vi "PhXP Settings Storage.vi"(6 "Set/Get(F)":bool, 8 "Error In":errorcluster, 10 "Variant Data in":variant, 11 "Settings List":T12) -> (0 "Error Out":errorcluster, 2 "Variant Data out":variant)   [LabVIEW 2019]
uses:
  Phasor Explorer Detector Parameters.ctl
  Phasor Explorer Gate Parameters.ctl
  Gate Type.ctl
  Phasor Explorer Decay Parameters.ctl
  IRF Model.ctl
  Phasor Explorer Phasor Parameters.ctl
  Phasor Calculation Type.ctl
  SEPL Type.ctl
  Phasor Explorer Display Parameters.ctl
  Type of Series.ctl
  Phasor Explorer Settings List.ctl
panel:
  in  "Parameter Tabs":T1(tab)=enum."Gates"
  in  "Phasor Explorer Display Parameters":T2={"# Points"=1000, "Ramp Type"=enum."Logarithmic", "Type of Series"=enum."1-Exp Decays", "Min tau"=1.0000000000000002e-12, "Max tau"=1.0000000000000001e-07, "Include 0"=FALSE, "Include Infinity"=FALSE} {"Min tau" min=0.0; "Max tau" min=0.0; "# Points" min=1 step=1}
  in  "f*":dbl[unit]=80000000.0 format="%#_5g"
  in  "tau*":dbl[unit]=1.9894367886486918e-09 format="%#_5g"
  in  "Phasor Explorer Phasor Parameters":T4={"Harmonic frequency"=80000000.0, "Use f* = 1/D Frequency"=FALSE, "Calibrated Phasor"=FALSE, "Calibration Lifetime"=1e-09, "Phasor Calculation"=enum."Direct Sum", "SEPL Type"=enum."UC", "# Gates"=1.0, "Square Gate Width"=1e-09, "Show Ticks"=FALSE} {"Square Gate Width" min=0.0; "# Gates" min=0.0; "Calibration Lifetime" min=0.0; "Harmonic frequency" min=0.0}
  in  "Phasor Explorer Decay Parameters":T7={"Lifetime"=3.0000000000000004e-09, "IRF Offset"=0.0, "IRF Period"=1.2500000000000001e-08, "Normalized Decays"=FALSE, "IRF Model"=enum."Dirac", "IRF Parameter 1"=0.0} {"Lifetime" min=0.0; "IRF Period" min=0.0}
  in  "Phasor Explorer Gate Parameters":T9={"First Gate Start"=0.0, "Use Gate Center"=FALSE, "Gate Width"=0.0, "Gate Step"=1.785714285714286e-09, "# Gates"=7.0, "Gate Type"=enum."Square", "Edge Width"=0.0, "Top Slope"=0.0, "Reversed Sawtooth?"=FALSE, "Analytical Computation"=FALSE, "Integration"=enum."Item 0", "Tolerance"=1.0, "# Steps"=1.0, "Type of User-defined Function"=enum."Gate", "Use Gate Step"=FALSE} {"# Steps" min=0.0; "Tolerance" min=0.0; "Top Slope" min=0.0; "Edge Width" min=0.0; "First Gate Start" format="%#_4g"; "Gate Step" min=0.0 format="%#_4g"; "# Gates" min=1.0 step=1.0; "Gate Width" min=0.0 format="%#_4g"}
  in  "Phasor Explorer Detector Parameters":T11={"Frames/Image"=0, "Gates/Frame"=1, "Bits/Frame"=1, "Multiplicity"=0, "Incident Signal"=0.0, "Poisson Signal"=FALSE} {"Frames/Image" min=1; "Multiplicity" min=0; "Bits/Frame" min=1; "Gates/Frame" min=1}
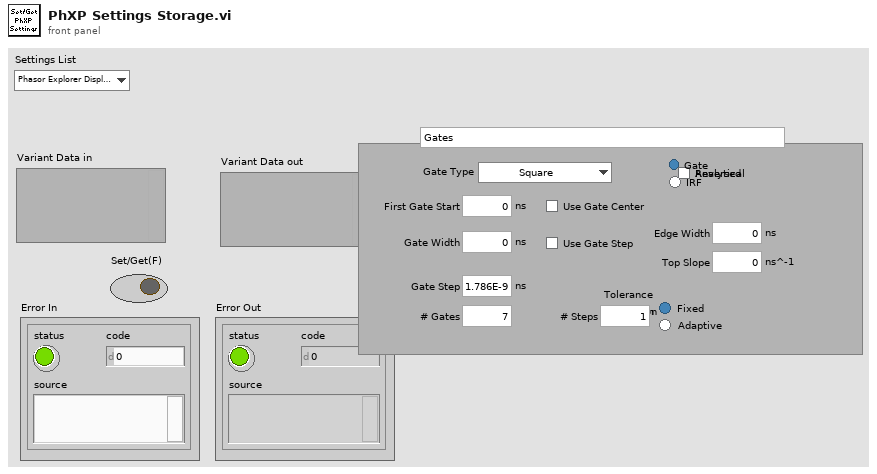
[diagram p1: front panel]
types:
  T1 = enum32{"Display", "Phasor", "Decay", "Gates", "Detector"}
  T2 = typedef "Phasor Explorer Display Parameters.ctl" = cluster{"# Points":i32, "Ramp Type":enum16{"Linear", "Logarithmic"}, "Type of Series":T3, "Min tau":dbl[unit], "Max tau":dbl[unit], "Include 0":bool, "Include Infinity":bool}
  T3 = typedef "Type of Series.ctl" = enum16{"1-Exp Decays", "Linear Combination of 1-Exp"}
  T4 = typedef "Phasor Explorer Phasor Parameters.ctl" = cluster{"Harmonic frequency":dbl[unit], "Use f* = 1/D Frequency":bool, "Calibrated Phasor":bool, "Calibration Lifetime":dbl[unit], "Phasor Calculation":T5, "SEPL Type":T6, "# Gates":dbl, "Square Gate Width":dbl[unit], "Show Ticks":bool}
  T5 = typedef "Phasor Calculation Type.ctl" = enum16{"Direct Sum", "Analytical Formula"}
  T6 = typedef "SEPL Type.ctl" = enum16{"UC", "L_N", "L_N[W]"}
  T7 = typedef "Phasor Explorer Decay Parameters.ctl" = cluster{"Lifetime":dbl[unit], "IRF Offset":dbl[unit], "IRF Period":dbl[unit], "Normalized Decays":bool, "IRF Model":T8, "IRF Parameter 1":dbl[unit]}
  T8 = typedef "IRF Model.ctl" = enum16{"Dirac", "Exponential"}
  T9 = typedef "Phasor Explorer Gate Parameters.ctl" = cluster{"First Gate Start":dbl[unit], "Use Gate Center":bool, "Gate Width":dbl[unit], "Gate Step":dbl[unit], "# Gates":dbl, "Gate Type":T10, "Edge Width":dbl[unit], "Top Slope":dbl[unit], "Reversed Sawtooth?":bool, "Analytical Computation":bool, "Integration":enum32{"Item 0", "Item 1"}, "Tolerance":dbl, "# Steps":dbl, "Type of User-defined Function":enum32{"Gate", "IRF"}, "Use Gate Step":bool}
  T10 = typedef "Gate Type.ctl" = enum16{"Square", "Finite Edge Square", "Finite Edge, Tilted Top Square", "Triangle", "Sawtooth", "User-defined"}
  T11 = typedef "Phasor Explorer Detector Parameters.ctl" = cluster{"Frames/Image":i32, "Gates/Frame":i32, "Bits/Frame":i32, "Multiplicity":i32, "Incident Signal":dbl, "Poisson Signal":bool}
  T12 = typedef "Phasor Explorer Settings List.ctl" = enum16{"Phasor Explorer Display Parameters", "Phasor Explorer Phasor Parameters", "Phasor Explorer Decay & IRF Parameters", "Phasor Explorer Gate Parameters", "Phasor Explorer Detector Parameters", "f*", "tau*"}
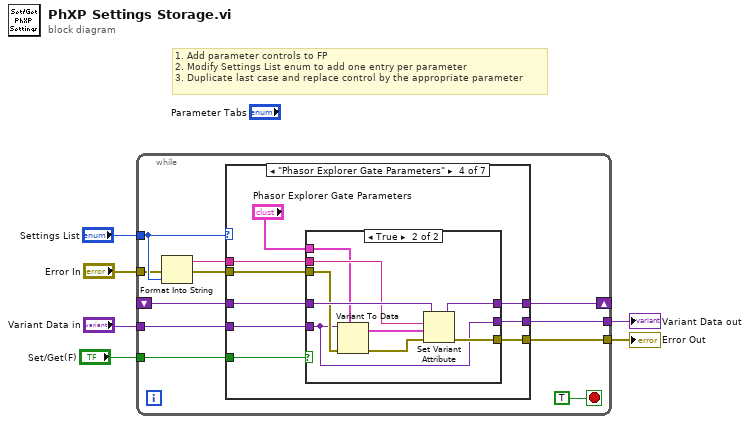
[diagram p0: block diagram]
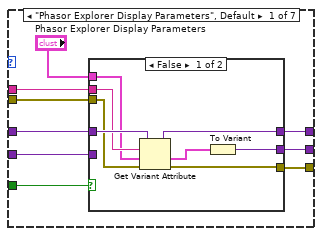
[diagram p2: hidden frame]
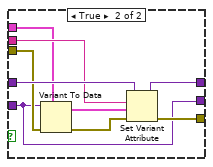
[diagram p3: hidden frame]
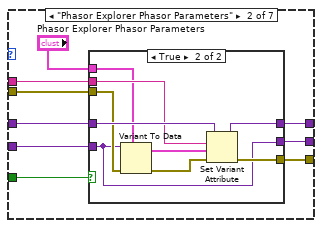
[diagram p4: hidden frame]
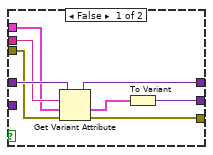
[diagram p5: hidden frame]
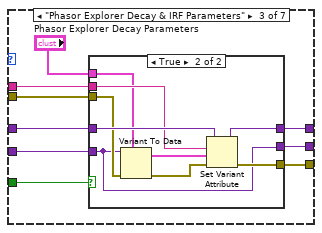
[diagram p6: hidden frame]
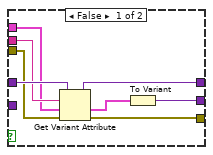
[diagram p7: hidden frame]
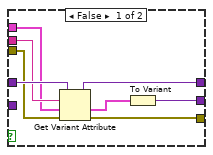
[diagram p8: hidden frame]
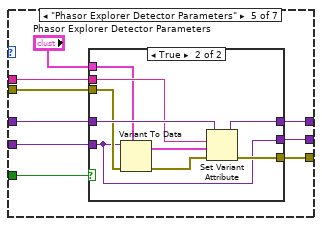
[diagram p9: hidden frame]
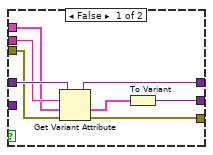
[diagram p10: hidden frame]
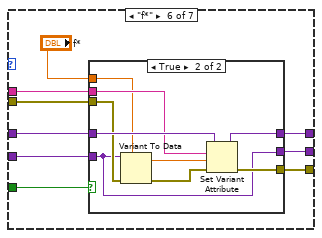
[diagram p11: hidden frame]
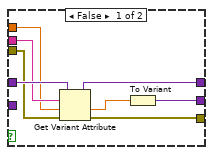
[diagram p12: hidden frame]
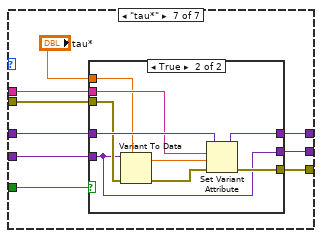
[diagram p13: hidden frame]
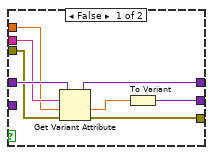
[diagram p14: hidden frame]
diagram:
  # "1. Add parameter controls to FP\n2. Modify Settings List enum to add one entry per parameter\n3. Duplicate last case and replace control by the appropriate parameter"
  n1 = while {
    tunnel: "Settings List" -> [w16]
    tunnel: "Error In" -> [w15]
    tunnel: "Set/Get(F)" -> [w14]
    shift-right: [w11] -> _
    shift-left: _ -> [w13]
    tunnel: "Variant Data in" -> [w9]
    tunnel: [w8] -> w2
    tunnel: [w7] -> w1
    stop <- TRUE stop-if-true
    n2 = Format Into String(error in=w15, w16) -> (resulting string=w12:string, error out=w10:errorcluster)  [unwired: 2 in]
    n3 = case shown="\"Phasor Explorer Gate Parameters\"" w16 {
      tunnel: w14 -> [w26 w52 w78 w104 w130 w156 w182]
      tunnel: w13 -> [w25 w51 w77 w103 w129 w155 w181]
      tunnel: w12 -> [w24 w50 w76 w102 w128 w154 w180]
      tunnel: [w23 w49 w75 w101 w127 w153 w179] -> w11
      tunnel: w10 -> [w22 w48 w74 w100 w126 w152 w178]
      tunnel: w9 -> [w21 w47 w73 w99 w125 w151 w177]
      tunnel: [w20 w46 w72 w98 w124 w150 w176] -> w8
      tunnel: [w19 w45 w71 w97 w123 w149 w175] -> w7
      frame "Phasor Explorer Display Parameters", Default {
        n4 = case shown="False" w26 {
          tunnel: w25 -> [w34 w43]
          tunnel: w24 -> [w33 w42]
          tunnel: [w31 w41] -> w23
          tunnel: "Phasor Explorer Display Parameters" -> [w28 w40]
          tunnel: w22 -> [w32 w39]
          tunnel: w21 -> [_ w35]
          tunnel: [w30 w36] -> w20
          tunnel: [w27 w35] -> w19
          frame False {
            n5 = Get Variant Attribute(Variant=w34, name=w33, default value (empty Variant)=w28, error in=w32) -> (duplicate Variant=w31:variant, value=w29:T2, error out=w30:errorcluster)  [unwired: 1 out]
            n6 = To Variant(anything=w29) -> (Variant=w27:variant)
          }
          frame True {
            n7 = Variant To Data(error in=w39, type=w40, Variant=w35) -> (data=w38:T2, error out=w37:errorcluster)
            n8 = Set Variant Attribute(Variant=w43, name=w42, value=w38, error in=w37) -> (Variant out=w41:variant, error out=w36:errorcluster)  [unwired: 1 out]
          }
        }
      }
      frame "Phasor Explorer Phasor Parameters" {
        n9 = case shown="True" w52 {
          tunnel: w51 -> [w60 w69]
          tunnel: w50 -> [w59 w68]
          tunnel: [w57 w67] -> w49
          tunnel: "Phasor Explorer Phasor Parameters" -> [w54 w66]
          tunnel: w48 -> [w58 w65]
          tunnel: w47 -> [_ w61]
          tunnel: [w56 w62] -> w46
          tunnel: [w53 w61] -> w45
          frame False {
            n10 = Get Variant Attribute(Variant=w60, name=w59, default value (empty Variant)=w54, error in=w58) -> (duplicate Variant=w57:variant, value=w55:T4, error out=w56:errorcluster)  [unwired: 1 out]
            n11 = To Variant(anything=w55) -> (Variant=w53:variant)
          }
          frame True {
            n12 = Variant To Data(error in=w65, type=w66, Variant=w61) -> (data=w64:T4, error out=w63:errorcluster)
            n13 = Set Variant Attribute(Variant=w69, name=w68, value=w64, error in=w63) -> (Variant out=w67:variant, error out=w62:errorcluster)  [unwired: 1 out]
          }
        }
      }
      frame "Phasor Explorer Decay & IRF Parameters" {
        n14 = case shown="True" w78 {
          tunnel: w77 -> [w86 w95]
          tunnel: w76 -> [w85 w94]
          tunnel: [w83 w93] -> w75
          tunnel: "Phasor Explorer Decay Parameters" -> [w80 w92]
          tunnel: w74 -> [w84 w91]
          tunnel: w73 -> [_ w87]
          tunnel: [w82 w88] -> w72
          tunnel: [w79 w87] -> w71
          frame False {
            n15 = Get Variant Attribute(Variant=w86, name=w85, default value (empty Variant)=w80, error in=w84) -> (duplicate Variant=w83:variant, value=w81:T7, error out=w82:errorcluster)  [unwired: 1 out]
            n16 = To Variant(anything=w81) -> (Variant=w79:variant)
          }
          frame True {
            n17 = Variant To Data(error in=w91, type=w92, Variant=w87) -> (data=w90:T7, error out=w89:errorcluster)
            n18 = Set Variant Attribute(Variant=w95, name=w94, value=w90, error in=w89) -> (Variant out=w93:variant, error out=w88:errorcluster)  [unwired: 1 out]
          }
        }
      }
      frame "Phasor Explorer Gate Parameters" {
        n19 = case shown="True" w104 {
          tunnel: w103 -> [w112 w121]
          tunnel: w102 -> [w111 w120]
          tunnel: [w109 w119] -> w101
          tunnel: "Phasor Explorer Gate Parameters" -> [w106 w118]
          tunnel: w100 -> [w110 w117]
          tunnel: w99 -> [_ w113]
          tunnel: [w108 w114] -> w98
          tunnel: [w105 w113] -> w97
          frame False {
            n20 = Get Variant Attribute(Variant=w112, name=w111, default value (empty Variant)=w106, error in=w110) -> (duplicate Variant=w109:variant, value=w107:T9, error out=w108:errorcluster)  [unwired: 1 out]
            n21 = To Variant(anything=w107) -> (Variant=w105:variant)
          }
          frame True {
            n22 = Variant To Data(error in=w117, type=w118, Variant=w113) -> (data=w116:T9, error out=w115:errorcluster)
            n23 = Set Variant Attribute(Variant=w121, name=w120, value=w116, error in=w115) -> (Variant out=w119:variant, error out=w114:errorcluster)  [unwired: 1 out]
          }
        }
      }
      frame "Phasor Explorer Detector Parameters" {
        n24 = case shown="True" w130 {
          tunnel: w129 -> [w138 w147]
          tunnel: w128 -> [w137 w146]
          tunnel: [w135 w145] -> w127
          tunnel: "Phasor Explorer Detector Parameters" -> [w132 w144]
          tunnel: w126 -> [w136 w143]
          tunnel: w125 -> [_ w139]
          tunnel: [w134 w140] -> w124
          tunnel: [w131 w139] -> w123
          frame False {
            n25 = Get Variant Attribute(Variant=w138, name=w137, default value (empty Variant)=w132, error in=w136) -> (duplicate Variant=w135:variant, value=w133:T11, error out=w134:errorcluster)  [unwired: 1 out]
            n26 = To Variant(anything=w133) -> (Variant=w131:variant)
          }
          frame True {
            n27 = Variant To Data(error in=w143, type=w144, Variant=w139) -> (data=w142:T11, error out=w141:errorcluster)
            n28 = Set Variant Attribute(Variant=w147, name=w146, value=w142, error in=w141) -> (Variant out=w145:variant, error out=w140:errorcluster)  [unwired: 1 out]
          }
        }
      }
      frame "f*" {
        n29 = case shown="True" w156 {
          tunnel: w155 -> [w164 w173]
          tunnel: w154 -> [w163 w172]
          tunnel: [w161 w171] -> w153
          tunnel: "f*" -> [w158 w170]
          tunnel: w152 -> [w162 w169]
          tunnel: w151 -> [_ w165]
          tunnel: [w160 w166] -> w150
          tunnel: [w157 w165] -> w149
          frame False {
            n30 = Get Variant Attribute(Variant=w164, name=w163, default value (empty Variant)=w158, error in=w162) -> (duplicate Variant=w161:variant, value=w159:dbl[unit], error out=w160:errorcluster)  [unwired: 1 out]
            n31 = To Variant(anything=w159) -> (Variant=w157:variant)
          }
          frame True {
            n32 = Variant To Data(error in=w169, type=w170, Variant=w165) -> (data=w168:dbl[unit], error out=w167:errorcluster)
            n33 = Set Variant Attribute(Variant=w173, name=w172, value=w168, error in=w167) -> (Variant out=w171:variant, error out=w166:errorcluster)  [unwired: 1 out]
          }
        }
      }
      frame "tau*" {
        n34 = case shown="True" w182 {
          tunnel: w181 -> [w190 w199]
          tunnel: w180 -> [w189 w198]
          tunnel: [w187 w197] -> w179
          tunnel: "tau*" -> [w184 w196]
          tunnel: w178 -> [w188 w195]
          tunnel: w177 -> [_ w191]
          tunnel: [w186 w192] -> w176
          tunnel: [w183 w191] -> w175
          frame False {
            n35 = Get Variant Attribute(Variant=w190, name=w189, default value (empty Variant)=w184, error in=w188) -> (duplicate Variant=w187:variant, value=w185:dbl[unit], error out=w186:errorcluster)  [unwired: 1 out]
            n36 = To Variant(anything=w185) -> (Variant=w183:variant)
          }
          frame True {
            n37 = Variant To Data(error in=w195, type=w196, Variant=w191) -> (data=w194:dbl[unit], error out=w193:errorcluster)
            n38 = Set Variant Attribute(Variant=w199, name=w198, value=w194, error in=w193) -> (Variant out=w197:variant, error out=w192:errorcluster)  [unwired: 1 out]
          }
        }
      }
    }
  }
  "Error Out" <- w2
  "Variant Data out" <- w1
